vi "Close.vi"(8 "error in (no error)":errorcluster, 11 "Huber Settings":T1) -> (0 "error out":errorcluster, 3 "Huber Settings":T1)   [LabVIEW 2018, in "Huber Unistat 410 TCU.lvlib"]
uses:
  Huber Unistat 410 TCU.lvlib
  Huber Unistat 410 Settings.ctl
panel:
  in  "Internal?":bool
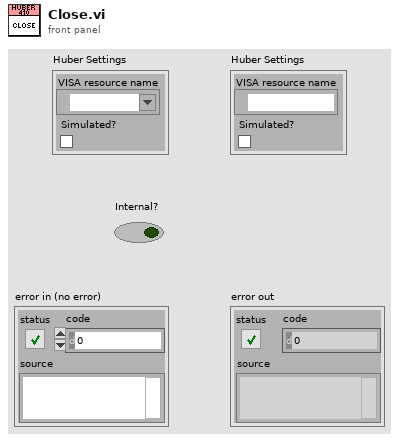
[diagram p1: front panel]
types:
  T1 = typedef "Huber Unistat 410 TCU.lvlib/Huber Unistat 410 Settings.ctl" = cluster{"VISA resource name":refnum<visa-resource-name>, "Simulated?":bool}
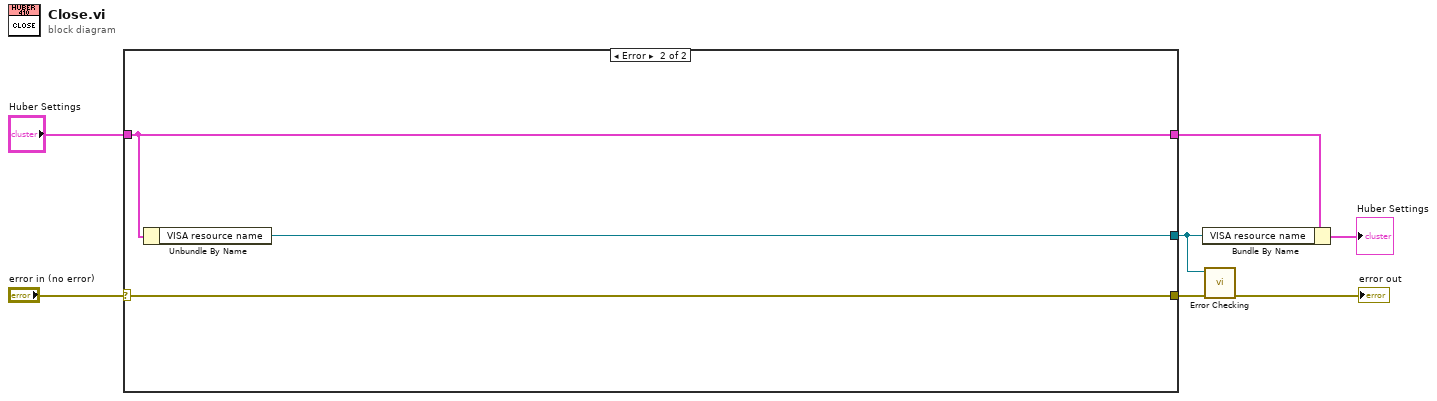
[diagram p0: block diagram]
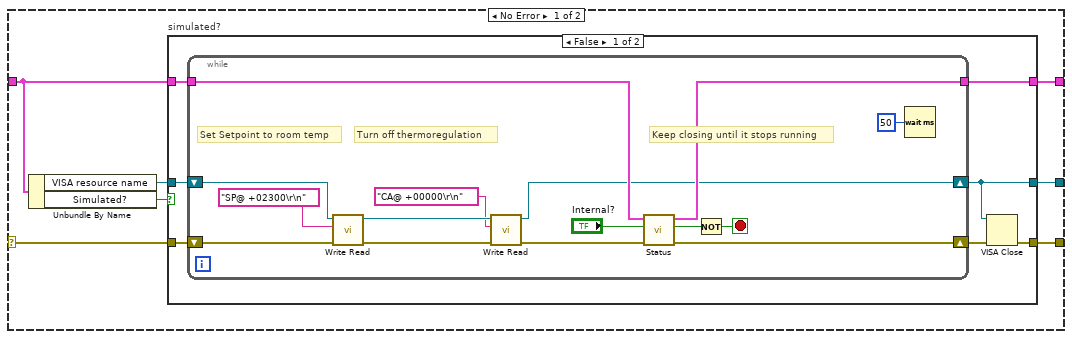
[diagram p2: hidden frame]
diagram:
  n1 = case shown="Error" "error in (no error)" {
    selector: "error in (no error)" -> [w12 w42]
    tunnel: [w13 w42] -> w6
    tunnel: "Huber Settings" -> [w9 w40]
    tunnel: [w10 w41] -> w4
    tunnel: [w8 w40] -> w3
    frame No Error {
      n2 = Unbundle By Name(w9) -> ("VISA resource name"=w11:refnum<visa-resource-name>, "Simulated?"=w14:bool)
      n3 = case "simulated?" shown="False" w14 {
        tunnel: [w19 w39] -> w13
        tunnel: w11 -> [w18 w38]
        tunnel: w12 -> [w21 w39]
        tunnel: [w17 w38] -> w10
        tunnel: w9 -> [w16 w37]
        tunnel: [w15 w37] -> w8
        frame False {
          n4 = while {
            shift-right: [w34] -> w20
            shift-left: w21 -> [w29]
            shift-right: [w27] -> w17
            shift-left: w18 -> [w31]
            tunnel: w16 -> [w35]
            tunnel: [w32] -> w15
            stop <- w36 stop-if-true
            # "Turn off thermoregulation"
            # "Set Setpoint to room temp"
            # "Keep closing until it stops running"
            n5 = call "Write Read.vi"("error in (no error)"=w29, "write string"="SP@ +02300\r\n" ("string"), "VISA Refnum in"=w31) -> ("error out"=w26:errorcluster, "VISA Refnum out"=w28:refnum<visa-resource-name>)  [unwired: 6 in, 1 out]
            n6 = call "Write Read.vi"("error in (no error)"=w26, "write string"="CA@ +00000\r\n" ("string"), "VISA Refnum in"=w28) -> ("error out"=w25:errorcluster, "VISA Refnum out"=w27:refnum<visa-resource-name>)  [unwired: 6 in, 1 out]
            n7 = call "Status.vi"("error in (no error)"=w25, "Internal?"="Internal?", "Huber Settings"=w35) -> ("error out"=w34:errorcluster, "Running"=w33:bool, "Huber Settings"=w32:T1)  [unwired: 4 in, 2 out]
            n8 = Not(x=w33) -> (.not. x?=w36:bool)
            n9 = Wait (ms)(milliseconds to wait=u32 50) -> ()  [unwired: 1 out]
          }
          n10 = VISA Close(VISA resource name=w17, error in (no error)=w20) -> (error out=w19:errorcluster)
        }
        frame True {
        }
      }
    }
    frame Error {
      n11 = Unbundle By Name(w40) -> ("VISA resource name"=w41:refnum<visa-resource-name>)
    }
  }
  n12 = Bundle By Name(cluster=w3, "VISA resource name"=w4) -> (→"Huber Settings":T1)
  n13 = call "Error Checking.vi"("error in (no error)"=w6, "VISA resource name"=w4) -> ("error out"=→"error out":errorcluster)  [unwired: 7 in, 2 out]
